vi "Get Acquired Data.vi"(5 "size":u32) -> (1 "arr 2":i32[][](array[numeric]), 2 "function return":u32)   [LabVIEW 2018, in "AndorSDK.lvlib"]
doc: "EXPNETTYPE unsigned int WINAPI GetAcquiredData(at_32 * arr, unsigned long size);"
uses:
  AndorSDK.lvlib
  ATMCD32D.dll
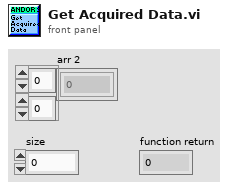
[diagram p1: front panel]
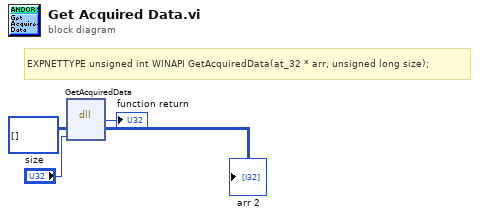
[diagram p0: block diagram]
diagram:
  # "EXPNETTYPE unsigned int WINAPI GetAcquiredData(at_32 * arr, unsigned long size);"
  n1 = dll-call lib="PTH2babs E\nPersönliches02 - Arbeit03-HiwijobsLabviewCodelibANDOR\tAndor SDK\nATMCD32D.*" fn="GetAcquiredData"("arr"=i32[][] [], "size"="size") -> ("return type"=→"function return":u32, "arr"=→"arr 2":i32[][])  [unwired: 4 in, 2 out]
